vi "Request Body.vi"(11 "Processing in":refnum<class "Processing.lvclass">) -> (3 "Processing out":refnum<class "Processing.lvclass">, 5 "Request Body":string)   [LabVIEW 2020, in "HTTP Server.lvlib" / "Processing.lvclass"]
uses:
  Processing.lvclass
  Processing.lvclass/Processing.ctl
  lv-http-util/HTTP Utils/Request/Request.lvclass
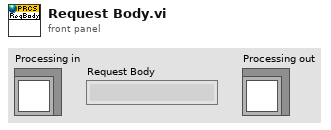
[diagram p1: front panel]
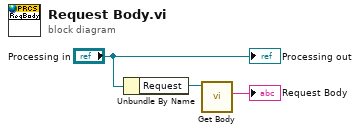
[diagram p0: block diagram]
diagram:
  n1 = Unbundle By Name("Processing in") -> ("Request"=w2:refnum<class "Request.lvclass">)
  n2 = call "Get Body.vi"("Request in"=w2) -> ("Body"=→"Request Body":string)  [unwired: 8 in, 2 out]
  "Processing out" <- "Processing in"
